vi "MotionMagicDrive_StateMachine.vi"(4 "Offset(Deg)":dbl format="%#_13g", 5 "High gear?":bool, 6 "Distance(Inches)":dbl format="%#_13g", 7 "Enable Vision":bool, 8 "error in (no error)":errorcluster, 9 "Y Axis":dbl, 10 "X Axis":dbl, 11 "Pod Drive in":refnum<class "Pod Drive.lvclass">) -> (0 "error out":errorcluster, 3 "Pod Drive out":refnum<class "Pod Drive.lvclass">)   [LabVIEW 2018, in "Drive.lvlib" / "Pod Drive.lvclass"]
doc: "This VI alows you to swich between motion magic GoTo and Closed Loop"
uses:
  Pod Drive.lvclass
  Mode.ctl
  Drive.lvclass
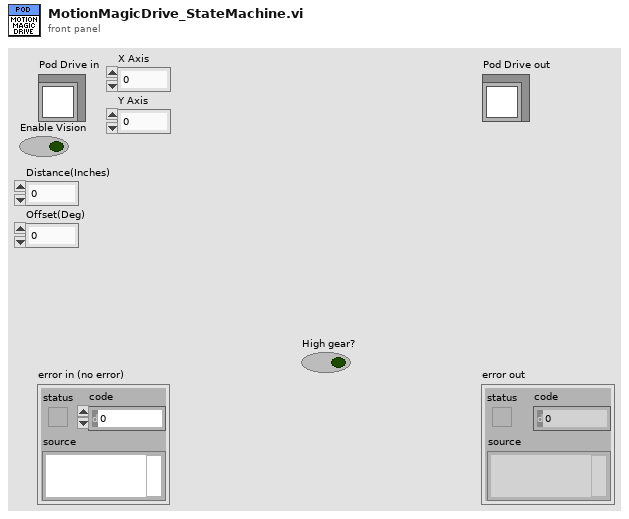
[diagram p1: front panel]
types:
  T1 = typedef "Drive.lvlib/Pod Drive.lvclass/Mode.ctl" = enum16{"ClosedLoop", "MotionMagic"}
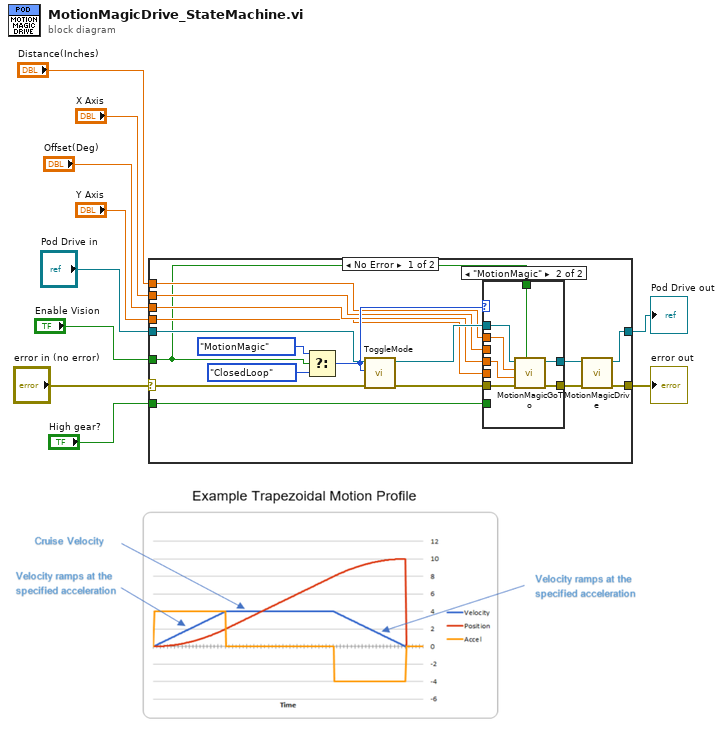
[diagram p0: block diagram]
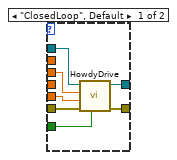
[diagram p2: hidden frame]
diagram:
  n1 = case shown="No Error" "error in (no error)" {
    selector: "error in (no error)" -> [w21 w42]
    tunnel: [w27 w42] -> w10
    tunnel: [w26 w43] -> w9
    tunnel: "Pod Drive in" -> [w18 w43]
    tunnel: "Enable Vision" -> [w11 _]
    tunnel: "Distance(Inches)" -> [w16 _]
    tunnel: "X Axis" -> [w15 _]
    tunnel: "Offset(Deg)" -> [w14 _]
    tunnel: "Y Axis" -> [w13 _]
    tunnel: "High gear?" -> [w12 _]
    frame No Error {
      n2 = Select(t=Mode."MotionMagic" ("ClosedLoopOrMotionMagic"), s=w11, f=Mode."ClosedLoop" ("ClosedLoopOrMotionMagic")) -> (s? t:f=w19:T1)
      n3 = call-dynamic "ToggleMode.vi"("error in (no error)"=w21, "Mode"=w19, "Pod Drive in"=w18) -> ("error out"=w20:errorcluster, "Pod Drive out"=w17:refnum<class "Pod Drive.lvclass">)  [unwired: 7 in]
      n4 = case shown="\"MotionMagic\"" w19 {
        tunnel: w17 -> [w34 w41]
        tunnel: [w33 w40] -> w25
        tunnel: w20 -> [w32 w39]
        tunnel: [w31 w38] -> w24
        tunnel: w16 -> [_ w36]
        tunnel: w14 -> [_ w37]
        tunnel: w13 -> [w29 _]
        tunnel: w15 -> [w30 _]
        tunnel: w12 -> [w28 _]
        tunnel: w11 -> [_ w35]
        frame "ClosedLoop", Default {
          n5 = call-dynamic "HowdyDrive.vi"("HighGear?"=w28, "error in (no error)"=w32, "Y"=w29, "X"=w30, "Pod Drive in"=w34) -> ("error out"=w31:errorcluster, "Pod Drive out"=w33:refnum<class "Pod Drive.lvclass">)  [unwired: 5 in]
        }
        frame "MotionMagic" {
          n6 = call "MotionMagicGoTo.vi"("Reset"=w35, "error in (no error)"=w39, "Offset(deg)"=w37, "Distance(in)"=w36, "Pod Drive in"=w41) -> ("error out"=w38:errorcluster, "Pod Drive out"=w40:refnum<class "Pod Drive.lvclass">)  [unwired: 4 in, 1 out]
        }
      }
      n7 = call-parent "MotionMagicDrive.vi"("error in (no error)"=w24, "Drive in"=w25) -> ("error out"=w27:errorcluster, "Drive out"=w26:refnum<class "Pod Drive.lvclass">)  [unwired: 8 in]
    }
    frame Error {
    }
  }
  "error out" <- w10
  "Pod Drive out" <- w9
